vi "onConfigurePeeling.vi"(8 "error in (no error)":errorcluster, 11 "Environment in":refnum<class "Environment.lvclass">) -> (0 "error out":errorcluster, 3 "Environment out":refnum<class "Environment.lvclass">)   [LabVIEW 2021, in "Bananas.lvlib" / "Environment.lvclass"]
uses:
  Environment.lvclass
  Environment.lvclass/Environment.ctl
  <vilib>/LabVIEW Open Source Project/Epoch Date & Time/epoch.UNIX/Epoch.UNIX.lvclass
  C:/Program Files (x86)/National Instruments/LabVIEW 2021/vi.lib/LabVIEW Open Source Project/Epoch Date & Time/epoch/Epoch.lvclass
  <vilib>/LabVIEW Open Source Project/Epoch Date & Time/Get Epoch Time.vi
  <vilib>/LabVIEW Open Source Project/Epoch Date & Time/epoch/Epoch.lvclass
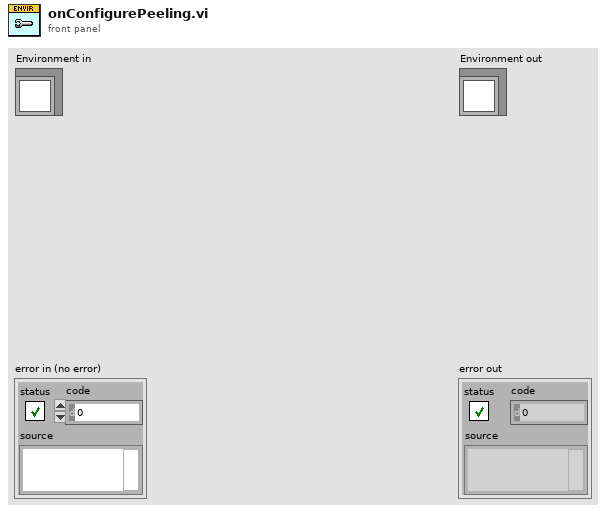
[diagram p1: front panel]
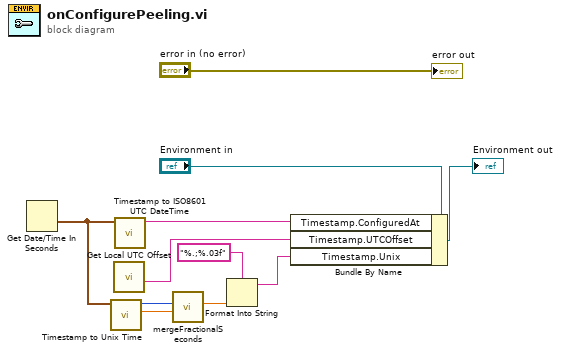
[diagram p0: block diagram]
diagram:
  n1 = Get Date/Time In Seconds() -> (seconds since 1Jan1904=w6:timestamp)
  n2 = call <vilib>:"Timestamp to Unix Time.vi"("Timestamp (now)"=w6) -> ("Fractional Second"=w4:dbl, "Unix Time (s)"=w5:i64)  [unwired: 9 in]
  n3 = call <vilib>:"Get Local UTC Offset.vi"() -> ("UTC Offset String"=w7:string)  [unwired: 10 in, 1 out]
  n4 = call <vilib>:"Timestamp to ISO8601 UTC DateTime.vi"("Timestamp (now)"=w6) -> ("ISO8601 UTC DateTime"=w9:string)  [unwired: 10 in]
  n5 = call <vilib>:"mergeFractionalSeconds.vi"("Fractional Second"=w4, "(Integer) Time (s)"=w5) -> ("(Float) Time (s)"=w3:dbl)  [unwired: 8 in, 1 out]
  n6 = Format Into String(format string="%.;%.03f", w3) -> (resulting string=w2:string)  [unwired: 2 in, 1 out]
  n7 = Bundle By Name(cluster="Environment in", "Timestamp.ConfiguredAt"=w9, "Timestamp.UTCOffset"=w7, "Timestamp.Unix"=w2) -> (→"Environment out":refnum<class "Environment.lvclass">)
  "error out" <- "error in (no error)"
